vi "Build Assert Variant.vi"(8 "error in (no error)":errorcluster, 10 "Assert Data":T1, 11 "Assert Variant in":variant) -> (0 "error out":errorcluster, 3 "Assert Variant out":variant)   [LabVIEW 2016, in "AssertEngine.lvlib" / "AssertEngine.lvclass"]
doc: "Builds up an assert configuration based on the Assert Data provided"
uses:
  AssertEngine.lvclass
  Log Assert/Assert Data.ctl
  Private Constants.vi
  AssertEngine.lvlib
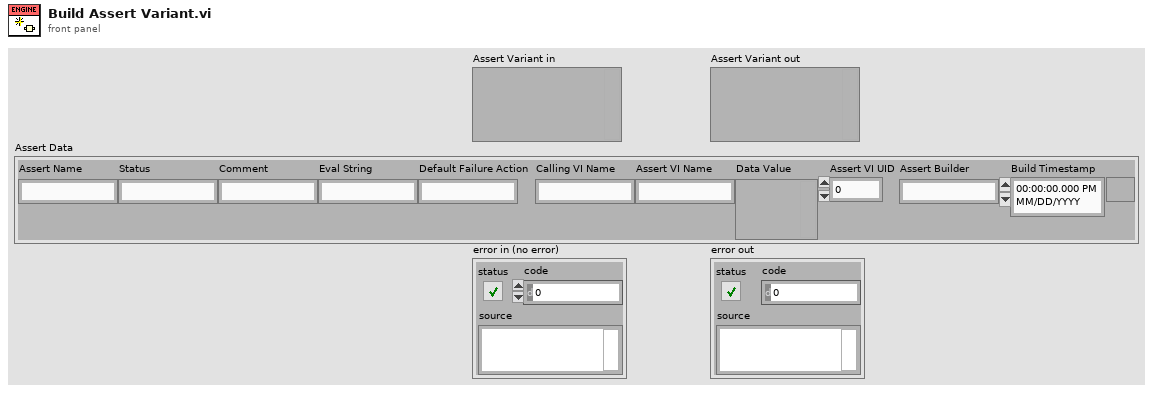
[diagram p1: front panel]
types:
  T1 = typedef "AssertEngine.lvlib/Assert Data.ctl" = cluster{"Assert Name":string, "Status":string, "Comment":string, "Eval String":string, "Default Failure Action":string, "Calling VI Name":string, "Assert VI Name":string, "Data Value":variant, "Assert VI UID":i32, "Assert Builder":string, "Build Timestamp":timestamp}
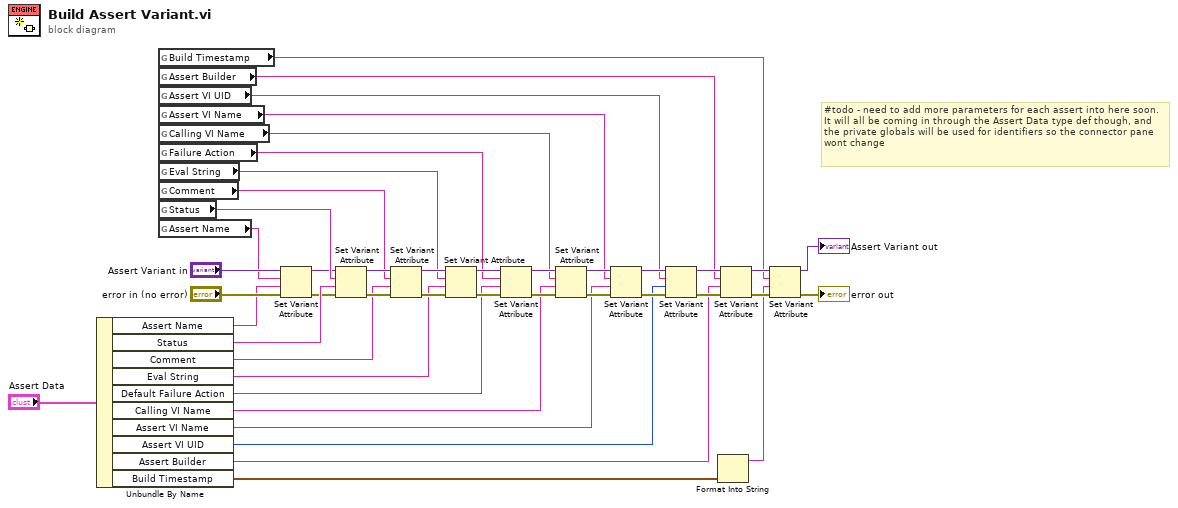
[diagram p0: block diagram]
diagram:
  # "#todo - need to add more parameters for each assert into here soon. It will all be coming in through the Assert Data type def though, and the private globals will be used for identifiers so the connector pane wont change"
  n1 = Unbundle By Name("Assert Data") -> ("Assert Name"=w23:string, "Status"=w43:string, "Comment"=w22:string, "Eval String"=w21:string, "Default Failure Action"=w20:string, "Calling VI Name"=w19:string, "Assert VI Name"=w18:string, "Assert VI UID"=w17:i32, "Assert Builder"=w8:string, "Build Timestamp"=w2:timestamp)
  n2 = global read "Private Constants.vi" "Build Timestamp"() -> (w3:string)
  n3 = global read "Private Constants.vi" "Assert Builder"() -> (w7:string)
  n4 = global read "Private Constants.vi" "Assert VI UID"() -> (w9:string)
  n5 = global read "Private Constants.vi" "Assert VI Name"() -> (w10:string)
  n6 = global read "Private Constants.vi" "Calling VI Name"() -> (w11:string)
  n7 = global read "Private Constants.vi" "Failure Action"() -> (w12:string)
  n8 = global read "Private Constants.vi" "Eval String"() -> (w13:string)
  n9 = global read "Private Constants.vi" "Comment"() -> (w14:string)
  n10 = global read "Private Constants.vi" "Status"() -> (w44:string)
  n11 = global read "Private Constants.vi" "Assert Name"() -> (w24:string)
  n12 = Set Variant Attribute(Variant="Assert Variant in", name=w24, value=w23, error in="error in (no error)") -> (Variant out=w25:variant, error out=w27:errorcluster)  [unwired: 1 out]
  n13 = Set Variant Attribute(Variant=w25, name=w44, value=w43, error in=w27) -> (Variant out=w36:variant, error out=w41:errorcluster)  [unwired: 1 out]
  n14 = Set Variant Attribute(Variant=w36, name=w14, value=w22, error in=w41) -> (Variant out=w35:variant, error out=w37:errorcluster)  [unwired: 1 out]
  n15 = Set Variant Attribute(Variant=w35, name=w13, value=w21, error in=w37) -> (Variant out=w33:variant, error out=w38:errorcluster)  [unwired: 1 out]
  n16 = Set Variant Attribute(Variant=w33, name=w12, value=w20, error in=w38) -> (Variant out=w32:variant, error out=w34:errorcluster)  [unwired: 1 out]
  n17 = Set Variant Attribute(Variant=w32, name=w11, value=w19, error in=w34) -> (Variant out=w29:variant, error out=w39:errorcluster)  [unwired: 1 out]
  n18 = Set Variant Attribute(Variant=w29, name=w10, value=w18, error in=w39) -> (Variant out=w28:variant, error out=w30:errorcluster)  [unwired: 1 out]
  n19 = Set Variant Attribute(Variant=w28, name=w9, value=w17, error in=w30) -> (Variant out=w15:variant, error out=w31:errorcluster)  [unwired: 1 out]
  n20 = Format Into String(w2) -> (resulting string=w1:string)  [unwired: 3 in, 1 out]
  n21 = Set Variant Attribute(Variant=w15, name=w7, value=w8, error in=w31) -> (Variant out=w5:variant, error out=w16:errorcluster)  [unwired: 1 out]
  n22 = Set Variant Attribute(Variant=w5, name=w3, value=w1, error in=w16) -> (Variant out=→"Assert Variant out":variant, error out=→"error out":errorcluster)  [unwired: 1 out]
